vi "SHAPE_getBestShapelets.vi"(10 "Number of Shapelets":i32, 11 "Population Notifier":refnum<notifier>) -> (3 "Population out":i32[][](array[numeric]))   [LabVIEW 2016, in "Shapelets Search (GA).lvlib"]
uses:
  Shapelets Search (GA).lvlib
  5. Features Optimization/_Optimal Frequency Bands Search/GA_core/GA_tPopulation.ctl
  5. Features Optimization/_Optimal Frequency Bands Search/GA_core/GeneticAlgorithm.lvlib
panel:
  out "Fitnesses":dbl[](array[numeric])
  # "This VI is a part of BCI Design library, http://www.ru-bci.org \nCopyright © 2020, Sotnikov Peter, All rights reserved. License: GNU GPLv3"
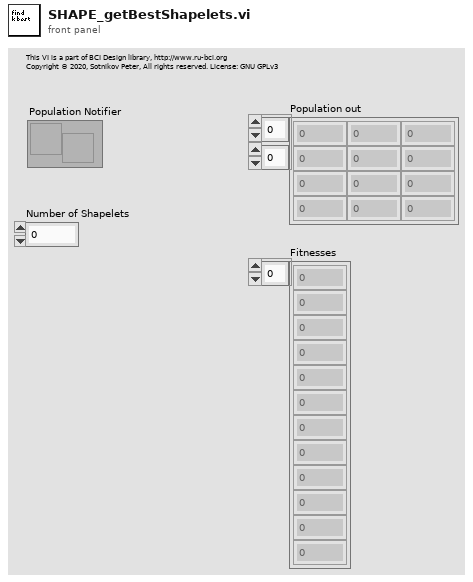
[diagram p1: front panel]
types:
  T1 = typedef "Optimal Frequency Bands Search.lvlib/GeneticAlgorithm.lvlib/GA_tPopulation.ctl" = cluster{"Population":i32[][], "Fitnesses":dbl[], "Sorted indices":i32[], "Ranks":i32[]}
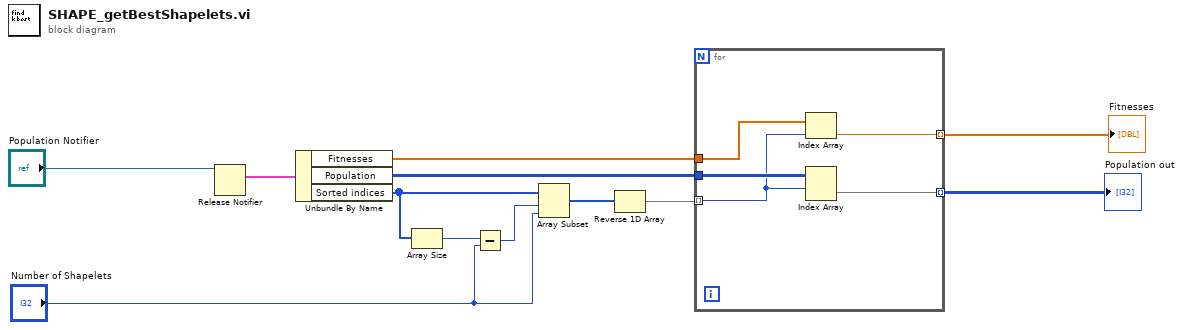
[diagram p0: block diagram]
diagram:
  n1 = Release Notifier(notifier="Population Notifier") -> (last notification=w11:T1)  [unwired: 2 in, 2 out]
  n2 = Unbundle By Name(w11) -> ("Fitnesses"=w5:dbl[], "Population"=w6:i32[][], "Sorted indices"=w10:i32[])
  n3 = Array Size(array=w10) -> (size(s)=w9:i32)
  n4 = Subtract(x=w9, y="Number of Shapelets") -> (x-y=w8:i32)
  n5 = Array Subset(array=w10, index=w8, length="Number of Shapelets") -> (w2:i32[])
  n6 = Reverse 1D Array(array=w2) -> (reversed array=w1:i32[])
  n7 = for {
    tunnel: w1 -> [w14] mode=indexing
    tunnel: w6 -> [w17]
    tunnel: [w16] -> w3 mode=indexing
    tunnel: w5 -> [w15]
    tunnel: [w13] -> w4 mode=indexing
    n8 = Index Array(array=w15, index=w14) -> (element=w13:dbl)
    n9 = Index Array(array=w17, index (row)=w14) -> (element=w16:i32[])  [unwired: 1 in]
  }
  "Population out" <- w3
  "Fitnesses" <- w4
